vi "Do.vi"(8 "error in (no error)":errorcluster, 10 "Actor in":refnum<class "Actor.lvclass">, 11 "Readout Msg":refnum<class "Readout Msg.lvclass">) -> (0 "error out":errorcluster, 2 "Actor out":refnum<class "Actor.lvclass">)   [LabVIEW 2021, in "BNT_ULx.lvlib" / "Readout Msg.lvclass"]
doc: "This VI delivers the message to the actor by calling the appropriate method(s) on the actor."
uses:
  Readout Msg.lvclass
  <vilib>/ActorFramework/Actor/Actor.lvclass
  BNT_ULx-MCSV/BNT_ULx-MCSV.lvclass
  C:/Program Files (x86)/National Instruments/LabVIEW 2021/vi.lib/ActorFramework/Actor/Actor.lvclass
  Readout Msg.lvclass/Readout Msg.ctl
  CSPP_Core/Messages/CSPP_AsyncCallbackMsg/CSPP_AsyncCallback Msg.lvclass
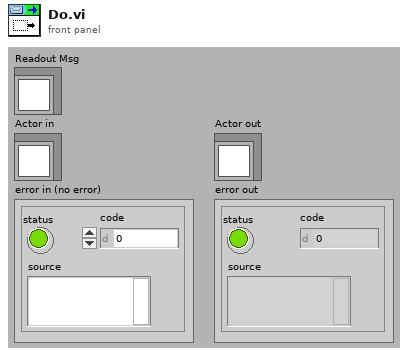
[diagram p1: front panel]
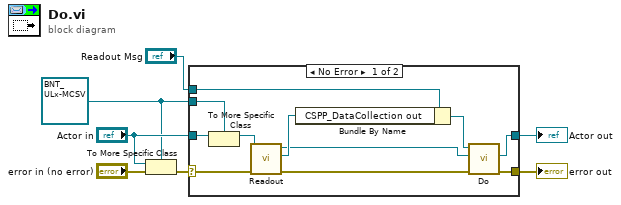
[diagram p0: block diagram]
diagram:
  w1 = refnum<class "BNT_ULx-MCSV.lvclass"> refnum ("BNT_ULx.lvlib:BNT_ULx-MCSV.lvclass")
  n1 = To More Specific Class(target class=w1, reference="Actor in", error in="error in (no error)") -> (error out=w6:errorcluster)  [unwired: 1 out]
  n2 = case shown="No Error" w6 {
    selector: w6 -> [w12 w20]
    tunnel: [w16 w20] -> w5
    tunnel: [w15 w19] -> w4
    tunnel: "Actor in" -> [w18 w19]
    tunnel: w1 -> [w17 _]
    tunnel: "Readout Msg" -> [w14 _]
    frame No Error {
      n3 = To More Specific Class ("To More Specific Class (internal)")(target class=w17, reference=w18) -> (specific class reference=w10:refnum<class "BNT_ULx-MCSV.lvclass">)  [unwired: 1 in, 1 out]
      n4 = call "Readout.vi"("Error In"=w12, "BNT_ULx-MCSV in"=w10) -> ("Error Out"=w11:errorcluster, "CSPP_DataCollection out"=w9:refnum<class "CSPP_DataCollection.lvclass">, "BNT_ULx-MCSV out"=w8:refnum<class "BNT_ULx-MCSV.lvclass">)  [unwired: 7 in]
      n5 = Bundle By Name ("Parent-Bundler")(cluster=w14, "CSPP_DataCollection out"=w9) -> (w13:refnum<class "Readout Msg.lvclass">)
      n6 = call-parent "Do.vi"("error in (no error)"=w11, "Actor in"=w8, "CSPP_AsyncCallback Msg"=w13) -> ("error out"=w16:errorcluster, "Actor out"=w15:refnum<class "Actor.lvclass">)  [unwired: 7 in]
    }
    frame Error {
    }
  }
  "error out" <- w5
  "Actor out" <- w4
